vi "GDSAPI_CreateMethods2.vi"(6 "PropertyMethodType":T1, 8 "error in (no error)":errorcluster, 10 "Methods":T2[](array[typedef]), 11 "ClassPath(*.lvclass)":path) -> (0 "error out":errorcluster, 3 "MethodsCreated":path[](array[path]))   [LabVIEW 2020]
doc: "This VI creates Methods in a class."
uses:
  <resource>/Framework/Providers/Open_GDS/ClassProviders/Common/String/GDSString_MethodDescriptionType.ctl
  <resource>/Framework/Providers/Open_GDS/ClassProviders/Common/CommonVIs/CommonVIs_AttributeType.ctl
  <resource>/Framework/Providers/Open_GDS/ClassProviders/Common/CommonVIs/CommonVIs_AttributeDataType.ctl
  <resource>/Framework/Providers/Open_GDS/ClassProviders/Common/String/GDSString_AccessScopeModifierType.ctl
  <resource>/Framework/Providers/Open_GDS/ClassProviders/Common/String/GDSString_ModifierType.ctl
  <resource>/Framework/Providers/Open_GDS/ClassProviders/Common/CommonVIs/CommonVIs_PropertyType.ctl
  <resource>/Framework/Providers/Open_GDS/API/GDSAPI_SubVIs/GDSAPI_PropertyMethodType.ctl
  <resource>/Framework/Providers/Open_GDS/API/GDSAPI_SubVIs/GDSAPI_MethodType.ctl
  <resource>/Framework/Providers/Open_GDS/ClassProviders/Provider_BaseClassInterface/CreateMethodData.ctl
  <resource>/Framework/Providers/Open_GDS/ClassProviders/Provider_EndevoGOOP300/GOOP300_SubVIs/GOOP300_MethodScopeType.ctl
  <resource>/Framework/Providers/Open_GDS/ClassProviders/Provider_LvNativeClass/ClassWriterNative_class/IconDetails.ctl
  <resource>/Framework/Providers/Open_GDS/ClassProviders/Provider_LvNativeClass/ClassWriterNative_class/IconSize.ctl
  <resource>/Framework/Providers/Open_GDS/ClassProviders/Provider_LvNativeClass/ClassWriterNative_class/ClassWriterNative.lvclass
  <resource>/Framework/Providers/Open_GDS/ClassProviders/Provider_BaseClassInterface/ClassWriter_class/ClassWriter.lvclass
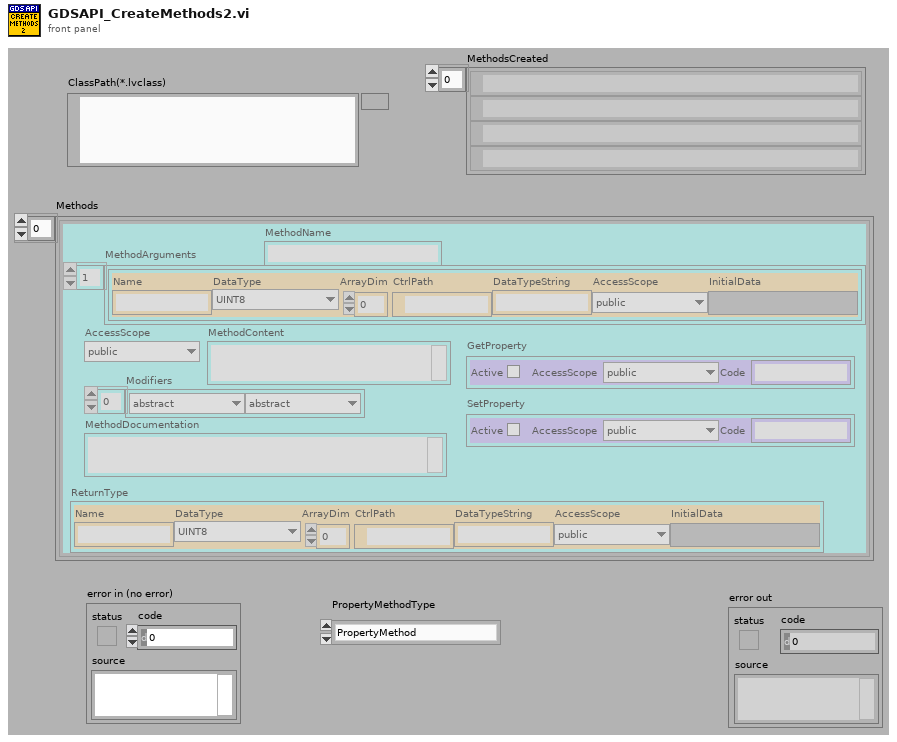
[diagram p1: front panel]
types:
  T1 = typedef "GDSAPI_PropertyMethodType.ctl" = enum16{"PropertyMethod", "PropertyNode"}
  T2 = typedef "GDSString_MethodDescriptionType.ctl" = cluster{"ReturnType":T3, "MethodName":string, "AccessScope":T5, "Modifiers":T6[], "MethodDocumentation":string, "MethodContent":string, "MethodArguments":T3[], "GetProperty":T7, "SetProperty":T7}
  T3 = typedef "CommonVIs_AttributeType.ctl" = cluster{"Name":string, "DataType":T4, "ArrayDim":i32, "CtrlPath":path, "DataTypeString":string, "AccessScope":T5, "InitialData":variant}
  T4 = typedef "CommonVIs_AttributeDataType.ctl" = enum16{"UINT8", "INT8", "UINT16", "INT16", "UINT32", "INT32", "UINT64", "INT64", "SGL", "DBL", "EXT", "CSG", "CDB", "CXT", "TimeStamp", "STRING", "PATH", "BOOL", "ENUM", "RefNum", "VIRefNum", "LabVIEW Class", "Cluster", "Variant", "TypeDef", "Waveform", "LabVIEW Object", "Other", "void"}
  T5 = typedef "GDSString_AccessScopeModifierType.ctl" = enum16{"public", "private", "protected", "internal"}
  T6 = typedef "GDSString_ModifierType.ctl" = enum16{"abstract", "static", "final", "synchronized", "strictfp", "async", "const", "event", "extern", "new", "native ", "override", "partial", "readonly", "sealed", "unsafe", "virtual", "volatile"}
  T7 = typedef "CommonVIs_PropertyType.ctl" = cluster{"Active":bool, "AccessScope":T5, "Code":string}
  T8 = typedef "GDSAPI_MethodType.ctl" = enum16{"Read Attribute", "Write Attribute", "Read & Write Attribute", "None Modifying Method", "Get Property", "Set Property", "Read Property", "Write Property", "Static Method", "Interface Method"}
  T9 = cluster{"AttributeNames":string[], "PropertyNode":bool, "FolderNames":string[]}
  T10 = typedef "ClassWriter.lvclass/CreateMethodData.ctl" = cluster{"MethodName":string, "RelativeMethodPath":path, "MethodDescription":string, "Scope/Visibility":T11, "MethodTemplateName":string, "IconOut":u8[][], "RelativeProjectClassPath":string, "OpenViAfterCreation":bool, "DynamicDispatchVi":bool, "ExtraCreateParameters":variant, "MustOverride":bool, "MustCallParent":bool, "IconDetails":T12, "AF-Option":variant, "TemplatePath":path}
  T11 = typedef "GOOP300_MethodScopeType.ctl" = enum16{"Use Parent Folder Scope", "Public", "Protected", "Private", "Community"}
  T12 = typedef "ClassWriterNative.lvclass/IconDetails.ctl" = cluster{"IconSize":T13, "ImageRows(32)":i32, "ConnectorPaneHeight":i32[]}
  T13 = typedef "ClassWriterNative.lvclass/IconSize.ctl" = enum16{"Full", "1 c-term high", "2 c-term high", "3 c-term high"}
  T14 = typedef "GDSLvCLass_ClassSettingsType.ctl" = cluster{"ClassProviderName":string, "ClassTemplateUsed":string, "ClassTemplateVersion":string, "ClassDescription":string, "PlugIns":T15[], "ConnectorPanePattern":string}
  T15 = typedef "GDSLvClass_PlugIn.ctl" = cluster{"Type":T16, "ID":string, "Version":string, "Path":path, "Name":string, "Data":variant}
  T16 = typedef "GDSLvClass_PlugInTypes.ctl" = enum16{"DesignPattern", "MethodTypes"}
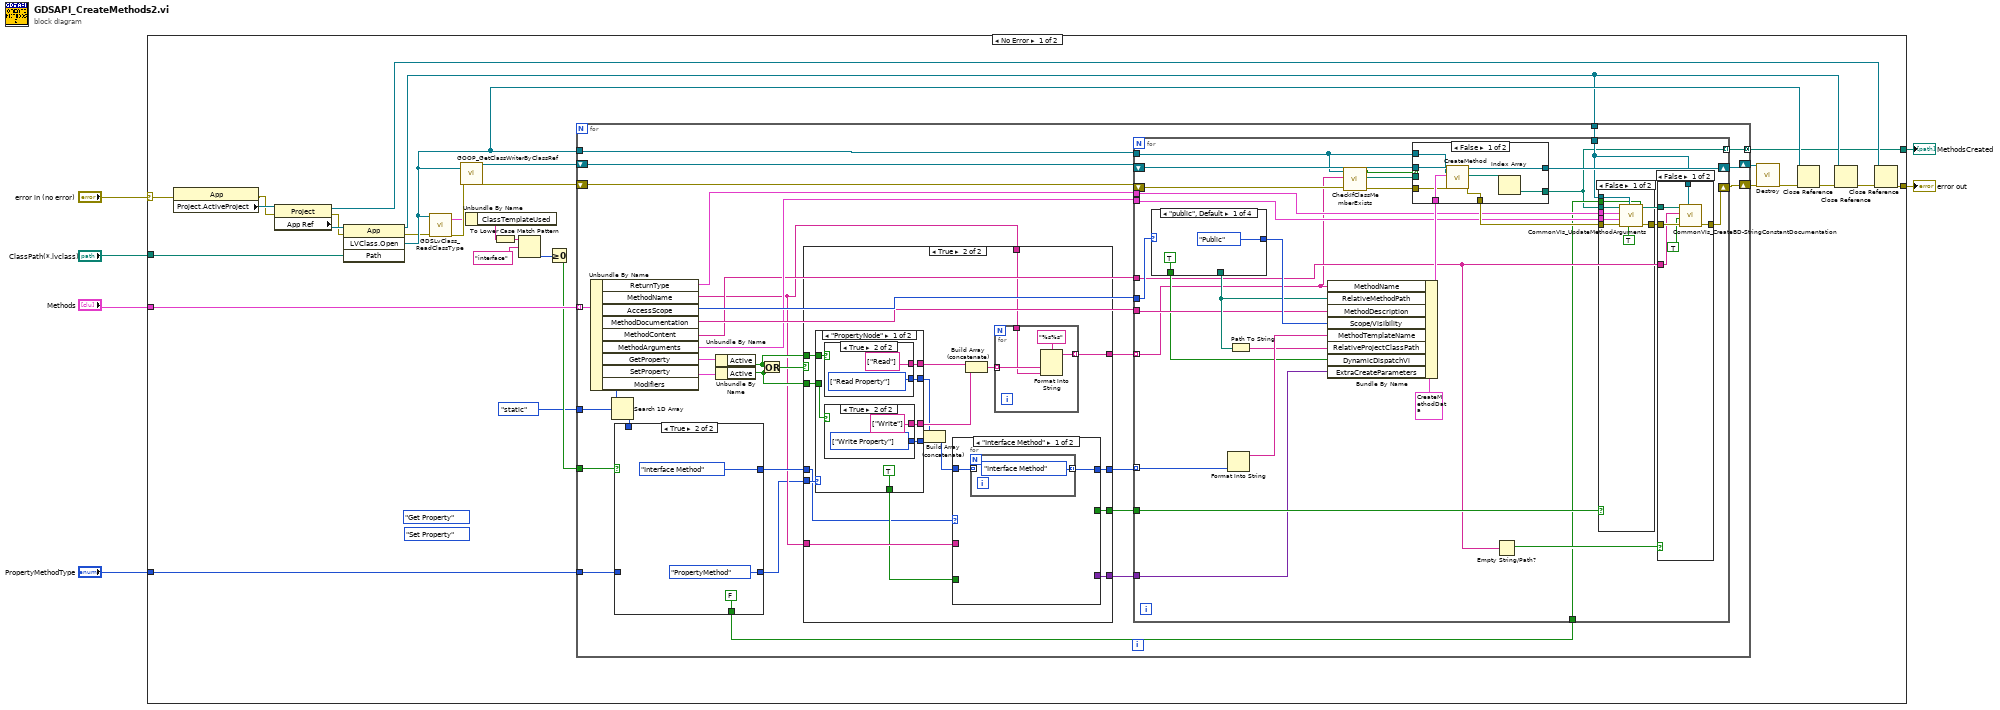
[diagram p0: block diagram]
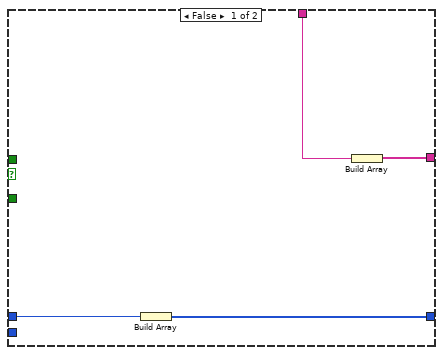
[diagram p2: hidden frame]
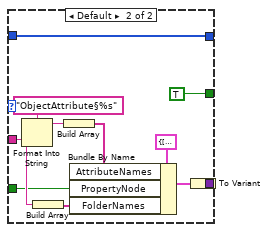
[diagram p3: hidden frame]
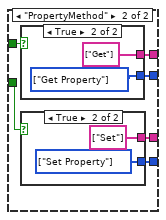
[diagram p6: hidden frame]
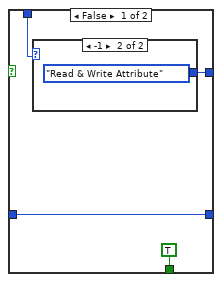
[diagram p9: hidden frame]
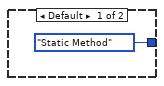
[diagram p10: hidden frame]
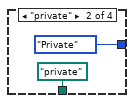
[diagram p14: hidden frame]
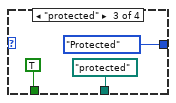
[diagram p15: hidden frame]
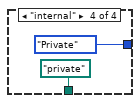
[diagram p16: hidden frame]
diagram:
  n1 = case shown="No Error" "error in (no error)" {
    selector: "error in (no error)" -> [w9 w202]
    tunnel: "ClassPath(*.lvclass)" -> [w35 _]
    tunnel: "Methods" -> [w34 _]
    tunnel: [w22 w202] -> w4
    tunnel: "PropertyMethodType" -> [w12 _]
    tunnel: [w7 _] -> w1
    frame No Error {
      (unwired) GDSAPI_MethodType."Set Property" ("MethodType")
      (unwired) GDSAPI_MethodType."Get Property" ("MethodType")
      n2 = property class="App"(error in=w9) -> (error out=w25:errorcluster, "Project.ActiveProject"=w28:refnum<vi>)  [unwired: 1 in, 1 out]
      n3 = property class="Project"(reference=w28, error in=w25) -> (reference out=w11:refnum<vi>, error out=w26:errorcluster, "App Ref"=w27:refnum<vi>)
      n4 = invoke class="App" method="LVClass.Open"(reference=w27, error in=w26, "Path"=w35) -> (reference out=w10:refnum<vi>, error out=w20:errorcluster, "LVClass.Open"=w21:refnum<vi>)  [unwired: 1 in, 1 out]
      n5 = call <resource>:"GDSLvClass_ReadClassType.vi"("Class Refnum In"=w21, "error in (no error)"=w20) -> ("ClassSettings"=w18:T14, "error out"=w19:errorcluster)  [unwired: 15 in, 1 out]
      n6 = call <resource>:"GOOP_GetClassWriterByClassRef.vi"("LVClassLibrary Refnum"=w21, "error in (no error)"=w19) -> ("ClassWriterNative.lvclass"=w29:refnum<class "ClassWriterNative.lvclass">, "error out"=w30:errorcluster)  [unwired: 16 in]
      n7 = Unbundle By Name(w18) -> ("ClassTemplateUsed"=w17:string)
      n8 = To Lower Case(string=w17) -> (all lower case string=w16:string)
      n9 = Match Pattern(string=w16, regular expression="interface") -> (offset past match=w14:i32)  [unwired: 1 in, 3 out]
      n10 = Greater Or Equal To 0?(x=w14) -> (x >= 0?=w13:bool)
      n11 = for {
        tunnel: w21 -> [w64]
        tunnel: w34 -> [w62] mode=indexing
        shift-right: [w59] -> w31
        shift-left: w30 -> [w65]
        shift-right: [w66] -> w32
        shift-left: w29 -> [w63]
        tunnel: w13 -> [w54]
        tunnel: w12 -> [w39]
        tunnel: w10 -> [w46]
        tunnel: GDSString_ModifierType."static" ("element") -> [w42]
        tunnel: [w36] -> w7 mode=concatenating
        n12 = Unbundle By Name(w62) -> ("ReturnType"=w58:T3, "MethodName"=w40:string, "AccessScope"=w61:T5, "MethodDocumentation"=w60:string, "MethodContent"=w45:string, "MethodArguments"=w57:T3[], "GetProperty"=w56:T7, "SetProperty"=w55:T7, "Modifiers"=w43:T6[])
        n13 = Search 1D Array(1D array=w43, element=w42) -> (index of element=w41:i32)  [unwired: 1 in]
        n14 = case shown="True" w54 {
          tunnel: [w130 GDSAPI_MethodType."Interface Method" ("MethodType")] -> w53
          tunnel: w41 -> [w129 _]
          tunnel: w39 -> [w128 _]
          tunnel: [w128 GDSAPI_PropertyMethodType."PropertyMethod" ("PropertyMethodType")] -> w38
          tunnel: [TRUE FALSE] -> w37
          frame False {
            n15 = case shown="-1" w129 {
              tunnel: [GDSAPI_MethodType."Static Method" ("MethodType") GDSAPI_MethodType."Read & Write Attribute" ("MethodType")] -> w130
              frame Default {
              }
              frame -1 {
              }
            }
          }
          frame True {
          }
        }
        n16 = Unbundle By Name(w56) -> ("Active"=w50:bool)
        n17 = Unbundle By Name(w55) -> ("Active"=w49:bool)
        n18 = Or(x=w50, y=w49) -> (x .or. y?=w51:bool)
        n19 = case shown="True" w51 {
          tunnel: w53 -> [w70 w74]
          tunnel: [w69 w86] -> w52
          tunnel: w50 -> [_ w87]
          tunnel: w49 -> [_ w85]
          tunnel: w38 -> [_ w84]
          tunnel: w40 -> [w67 w79]
          tunnel: [_ w83] -> w48
          tunnel: [_ w82] -> w47
          tunnel: w40 -> [_ w81]
          tunnel: [w68 w78] -> w44
          frame False {
            n20 = Build Array(w70) -> (w69:T8[])
            n21 = Build Array(w67) -> (w68:string[])
          }
          frame True {
            n22 = case shown="\"PropertyNode\"" w84 {
              tunnel: w87 -> [w112 w122]
              tunnel: w85 -> [w111 w121]
              tunnel: [w110 w120] -> w72
              tunnel: [w109 w119] -> w73
              tunnel: [TRUE _] -> w80
              tunnel: [w107 w118] -> w76
              tunnel: [w106 w117] -> w75
              frame "PropertyNode" {
                n23 = case shown="True" w112 {
                  tunnel: [_ w116] -> w110
                  tunnel: [_ string[] ["Read"]] -> w107
                  frame False {
                  }
                  frame True {
                    w116 = T8[] [enum."Read Property"] items=["Read Attribute", "Write Attribute", "Read & Write Attribute", "None Modifying Method", "Get Property", "Set Property", "Read Property", "Write Property", "Static Method", "Interface Method"]
                  }
                }
                n24 = case shown="True" w111 {
                  tunnel: [_ w114] -> w109
                  tunnel: [_ string[] ["Write"]] -> w106
                  frame False {
                  }
                  frame True {
                    w114 = T8[] [enum."Write Property"] items=["Read Attribute", "Write Attribute", "Read & Write Attribute", "None Modifying Method", "Get Property", "Set Property", "Read Property", "Write Property", "Static Method", "Interface Method"]
                  }
                }
              }
              frame "PropertyMethod" {
                n25 = case shown="True" w122 {
                  tunnel: [_ w126] -> w120
                  tunnel: [_ string[] ["Get"]] -> w118
                  frame False {
                  }
                  frame True {
                    w126 = T8[] [enum."Get Property"] items=["Read Attribute", "Write Attribute", "Read & Write Attribute", "None Modifying Method", "Get Property", "Set Property", "Read Property", "Write Property", "Static Method", "Interface Method"]
                  }
                }
                n26 = case shown="True" w121 {
                  tunnel: [_ w124] -> w119
                  tunnel: [_ string[] ["Set"]] -> w117
                  frame False {
                  }
                  frame True {
                    w124 = T8[] [enum."Set Property"] items=["Read Attribute", "Write Attribute", "Read & Write Attribute", "None Modifying Method", "Get Property", "Set Property", "Read Property", "Write Property", "Static Method", "Interface Method"]
                  }
                }
              }
            }
            n27 = Build Array (concatenate)(w72, w73) -> (w71:T8[])
            n28 = case shown="\"Interface Method\"" w74 {
              tunnel: [w88 w92] -> w86
              tunnel: w71 -> [w89 w92]
              tunnel: [_ TRUE] -> w83
              tunnel: [_ w95] -> w82
              tunnel: w81 -> [_ w94]
              tunnel: w80 -> [_ w93]
              frame "Interface Method" {
                n29 = for {
                  tunnel: w89 -> [_] mode=indexing
                  tunnel: [GDSAPI_MethodType."Interface Method" ("MethodType")] -> w88 mode=indexing
                }
              }
              frame Default {
                n30 = Format Into String(format string="ObjectAttribute§%s", w94) -> (resulting string=w99:string)  [unwired: 2 in, 1 out]
                n31 = Build Array(w94) -> (w101:string[])
                n32 = Build Array(w99) -> (w100:string[])
                n33 = Bundle By Name(cluster=T9 {"AttributeNames"=[], "PropertyNode"=FALSE, "FolderNames"=[]}, "AttributeNames"=w100, "PropertyNode"=w93, "FolderNames"=w101) -> (w96:T9)
                n34 = To Variant(anything=w96) -> (Variant=w95:variant)
              }
            }
            n35 = Build Array (concatenate)(w76, w75) -> (w77:string[])
            n36 = for {
              tunnel: w77 -> [w105] mode=indexing
              tunnel: w79 -> [w104]
              tunnel: [w103] -> w78 mode=indexing
              n37 = Format Into String(format string="%s%s", w105, w104) -> (resulting string=w103:string)  [unwired: 2 in, 1 out]
            }
          }
        }
        n38 = for {
          tunnel: w64 -> [w141]
          tunnel: w61 -> [w159]
          tunnel: w60 -> [w156]
          tunnel: w52 -> [w151] mode=indexing
          tunnel: w58 -> [w153]
          tunnel: w57 -> [w152]
          shift-right: [w147] -> w59
          shift-left: w65 -> [w143]
          shift-right: [w165] -> w66
          shift-left: w63 -> [w164]
          tunnel: w48 -> [w150]
          tunnel: w47 -> [w149]
          tunnel: w46 -> [w146]
          tunnel: w45 -> [w145]
          tunnel: w44 -> [w138] mode=indexing
          tunnel: w37 -> [w137]
          tunnel: [w136] -> w36 mode=indexing
          n39 = case shown="\"public\", Default" w159 {
            tunnel: [GOOP300_MethodScopeType."Public" ("Scope/Visibility") GOOP300_MethodScopeType."Private" ("Scope/Visibility") GOOP300_MethodScopeType."Protected" ("Scope/Visibility") GOOP300_MethodScopeType."Private" ("Scope/Visibility")] -> w162
            tunnel: [_ path "private" ("RelativeMethodPath") path "protected" ("RelativeMethodPath") path "private" ("RelativeMethodPath")] -> w158
            tunnel: [TRUE _ TRUE _] -> w155
            frame "public", Default {
            }
            frame "private" {
            }
            frame "protected" {
            }
            frame "internal" {
            }
          }
          n40 = Format Into String(w151) -> (resulting string=w160:string)  [unwired: 3 in, 1 out]
          n41 = Path To String(path=w158) -> (string=w157:string)
          n42 = Bundle By Name(cluster=T10 {"MethodName"="", "RelativeMethodPath"=path "", "MethodDescription"="", "Scope/Visibility"=enum."Use Parent Folder Scope", "MethodTemplateName"="", "IconOut"=[], "RelativeProjectClassPath"="", "OpenViAfterCreation"=FALSE, "DynamicDispatchVi"=FALSE, "ExtraCreateParameters"=variant, "MustOverride"=FALSE, "MustCallParent"=FALSE, "IconDetails"={"IconSize"=enum."Full", "ImageRows(32)"=0, "ConnectorPaneHeight"=[]}, "AF-Option"=variant, "TemplatePath"=path ""} ("CreateMethodData"), "MethodName"=w138, "RelativeMethodPath"=w158, "MethodDescription"=w156, "Scope/Visibility"=w162, "MethodTemplateName"=w160, "RelativeProjectClassPath"=w157, "DynamicDispatchVi"=w155, "ExtraCreateParameters"=w149) -> (w161:T10)
          n43 = call <resource>:"CheckIfClassMemberExists.vi"("error in (no error)"=w143, "MethodName"=w138, "LVClassLibrary in"=w141) -> ("error out"=w142:errorcluster, "Path"=w139:path, "Exists"=w140:bool)  [unwired: 6 in]
          n44 = case shown="False" w140 {
            tunnel: [w173 w176] -> w165
            tunnel: w164 -> [w172 w176]
            tunnel: w161 -> [w171 _]
            tunnel: [w170 w175] -> w154
            tunnel: w142 -> [w169 w175]
            tunnel: w141 -> [w168 _]
            tunnel: [w166 w174] -> w136
            tunnel: w139 -> [_ w174]
            frame False {
              n45 = call-dynamic "CreateMethod.vi"("ClassWriterNative.lvclass"=w172, "ClassItemRefIn"=w168, "CreateMethodData"=w171, "error in (no error)"=w169) -> ("ClassWriterNative.lvclass 2"=w173:refnum<class "ClassWriterNative.lvclass">, "MethodPaths"=w167:path[], "error out"=w170:errorcluster)  [unwired: 12 in, 1 out]
              n46 = Index Array(array=w167) -> (element=w166:path)  [unwired: 1 in]
            }
            frame True {
            }
          }
          n47 = Empty String/Path?(string/path=w145) -> (empty?=w144:bool)
          n48 = case shown="False" w150 {
            tunnel: w136 -> [w191 _]
            tunnel: w154 -> [w190 w192]
            tunnel: [w189 w192] -> w148
            tunnel: w153 -> [w188 _]
            tunnel: w152 -> [w187 _]
            tunnel: w146 -> [w186 _]
            tunnel: w137 -> [w184 _]
            frame False {
              n49 = call <resource>:"CommonVIs_UpdateMethodArguments.vi"("CleanUpControls(True)"=w184, "Keep Existing Controls And Indicatores connected(False)"=TRUE, "App"=w186, "error in (no error)"=w190, "MethodArguments"=w187, "ReturnType"=w188, "VI Ref/Vi Path"=w191) -> ("error out"=w189:errorcluster)  [unwired: 4 in]
            }
            frame True {
            }
          }
          n50 = case shown="False" w144 {
            tunnel: w148 -> [w182 w183]
            tunnel: [w181 w183] -> w147
            tunnel: w136 -> [w180 _]
            tunnel: w146 -> [w179 _]
            tunnel: w145 -> [w177 _]
            frame False {
              n51 = call <resource>:"CommonVIs_CreateBD-StringConstantDocumentation.vi"("App"=w179, "error in (no error)"=w182, "Remove extra prefixed spaces on every row but keep indentation"=TRUE ("Remove extar prefixed spaces on every row but keep indentation"), "Documentation"=w177, "VI Ref/Vi Path"=w180) -> ("error out"=w181:errorcluster)  [unwired: 6 in]
            }
            frame True {
            }
          }
        }
      }
      n52 = call-dynamic "Destroy.vi"("ClassWriterNative"=w32, "error in (no error)"=w31) -> ("error out"=w33:errorcluster)  [unwired: 17 in]
      n53 = Close Reference(reference=w21, error in (no error)=w33) -> (error out=w24:errorcluster)
      n54 = Close Reference(reference=w10, error in (no error)=w24) -> (error out=w23:errorcluster)
      n55 = Close Reference(reference=w11, error in (no error)=w23) -> (error out=w22:errorcluster)
    }
    frame Error {
    }
  }
  "error out" <- w4
  "MethodsCreated" <- w1
